vi "MFC_PID_flow_new.vi"() -> ()   [LabVIEW 2021]
uses:
  OdorSensorArray/labview 2016 code/osa_global_save2.vi
  <vilib>/Utility/file.llb/Read From Spreadsheet File (DBL).vi
  <vilib>/measure/NI_MABase.lvlib
panel:
  in  "Stair interval (s)":u32=20
  out "Error U3-2 A0":string
  out "PID / flow":cluster{"Value Read":dbl, "Value Read":dbl}(graph)
  in  "Dilusion_lj2_DAC1":dbl step=0.1 format="%.4f"
  out "elapsed time":string="00:00:00.000"
  in  "MFC_sequence":path
  out "Array Size":i32
  out "Udate Array from File":sgl[](array[numeric])
  out "Error  PID_Save":string
  out "error write":errorcluster
  in  "Save file":bool
  in  "save data folder":path
  out "appended path":path
  out "AIN0":dbl format="%.6f"
  out "MFC I/O":cluster{"Value Read":dbl, "Value Read":dbl}(graph)
  out "AIN2":dbl format="%.6f"
  out "AIN1":dbl format="%.6f"
  in  "DAC0_type":enum16{"functional", "fixed", "read"}(ring)
  out "Waveform Chart":dbl(graph)
  in  "DAC0_fixed":dbl step=0.1 format="%.4f"
  out "Error DAC1,B":string
  out "error read":errorcluster
  in  "Background_DAC1":dbl step=0.1 format="%.4f"
  in  "Update Interval (ms)":u32=20
  out "Error_DAC0":string
  in  "Function":u16(ring) items=["Sine Wave", "Triangle Wave", "Square Wave", "Sawtooth Wave"]
  in  "Min Voltage":dbl=0.5 min=0.0 max=5.0 step=0.1 format="%.2f"
  in  "Max Voltage":dbl=4.5 min=0.0 max=5.0 step=0.1 format="%.2f"
  in  "Frequency (Hz)":dbl=1.0 step=0.1 format="%.3f"
  in  "Stop":bool
  # "Updates DAC0 at the specified update interval in order to build time series waveforms.  The\nupdate interval is set to 20 ms by default, but can be set lower based on the execution times\ndiscussed in Section 3.1 of the U3 User's Guide.  Uses the first found U3.\n\nWith a software timed application such as this, you might be able to reduce timing jitter (caused\nby the operating system) by increasing the priority of this process (labview.exe) in Windows\nTask Manager."
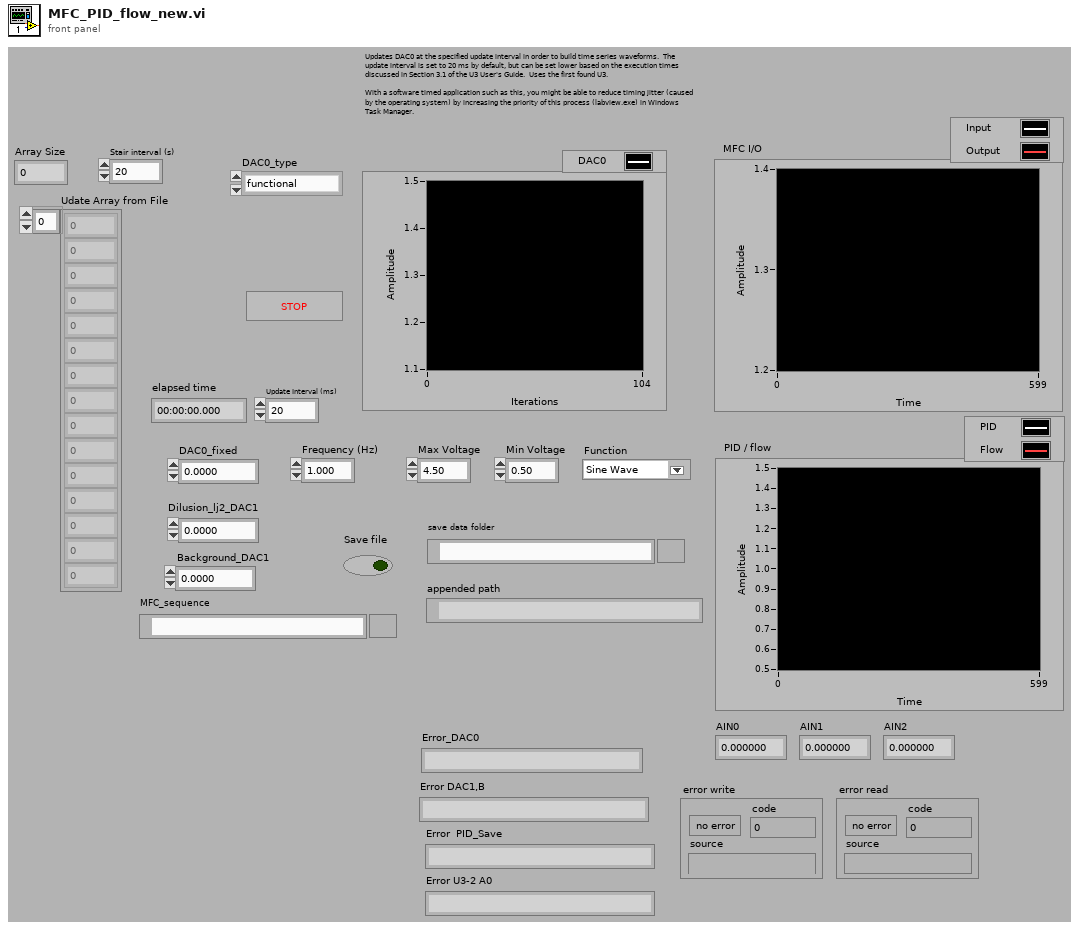
[diagram p1: front panel]
types:
  T1 = enum16{"open", "replace", "create", "open or create", "replace or create", "replace or create with confirmation"}
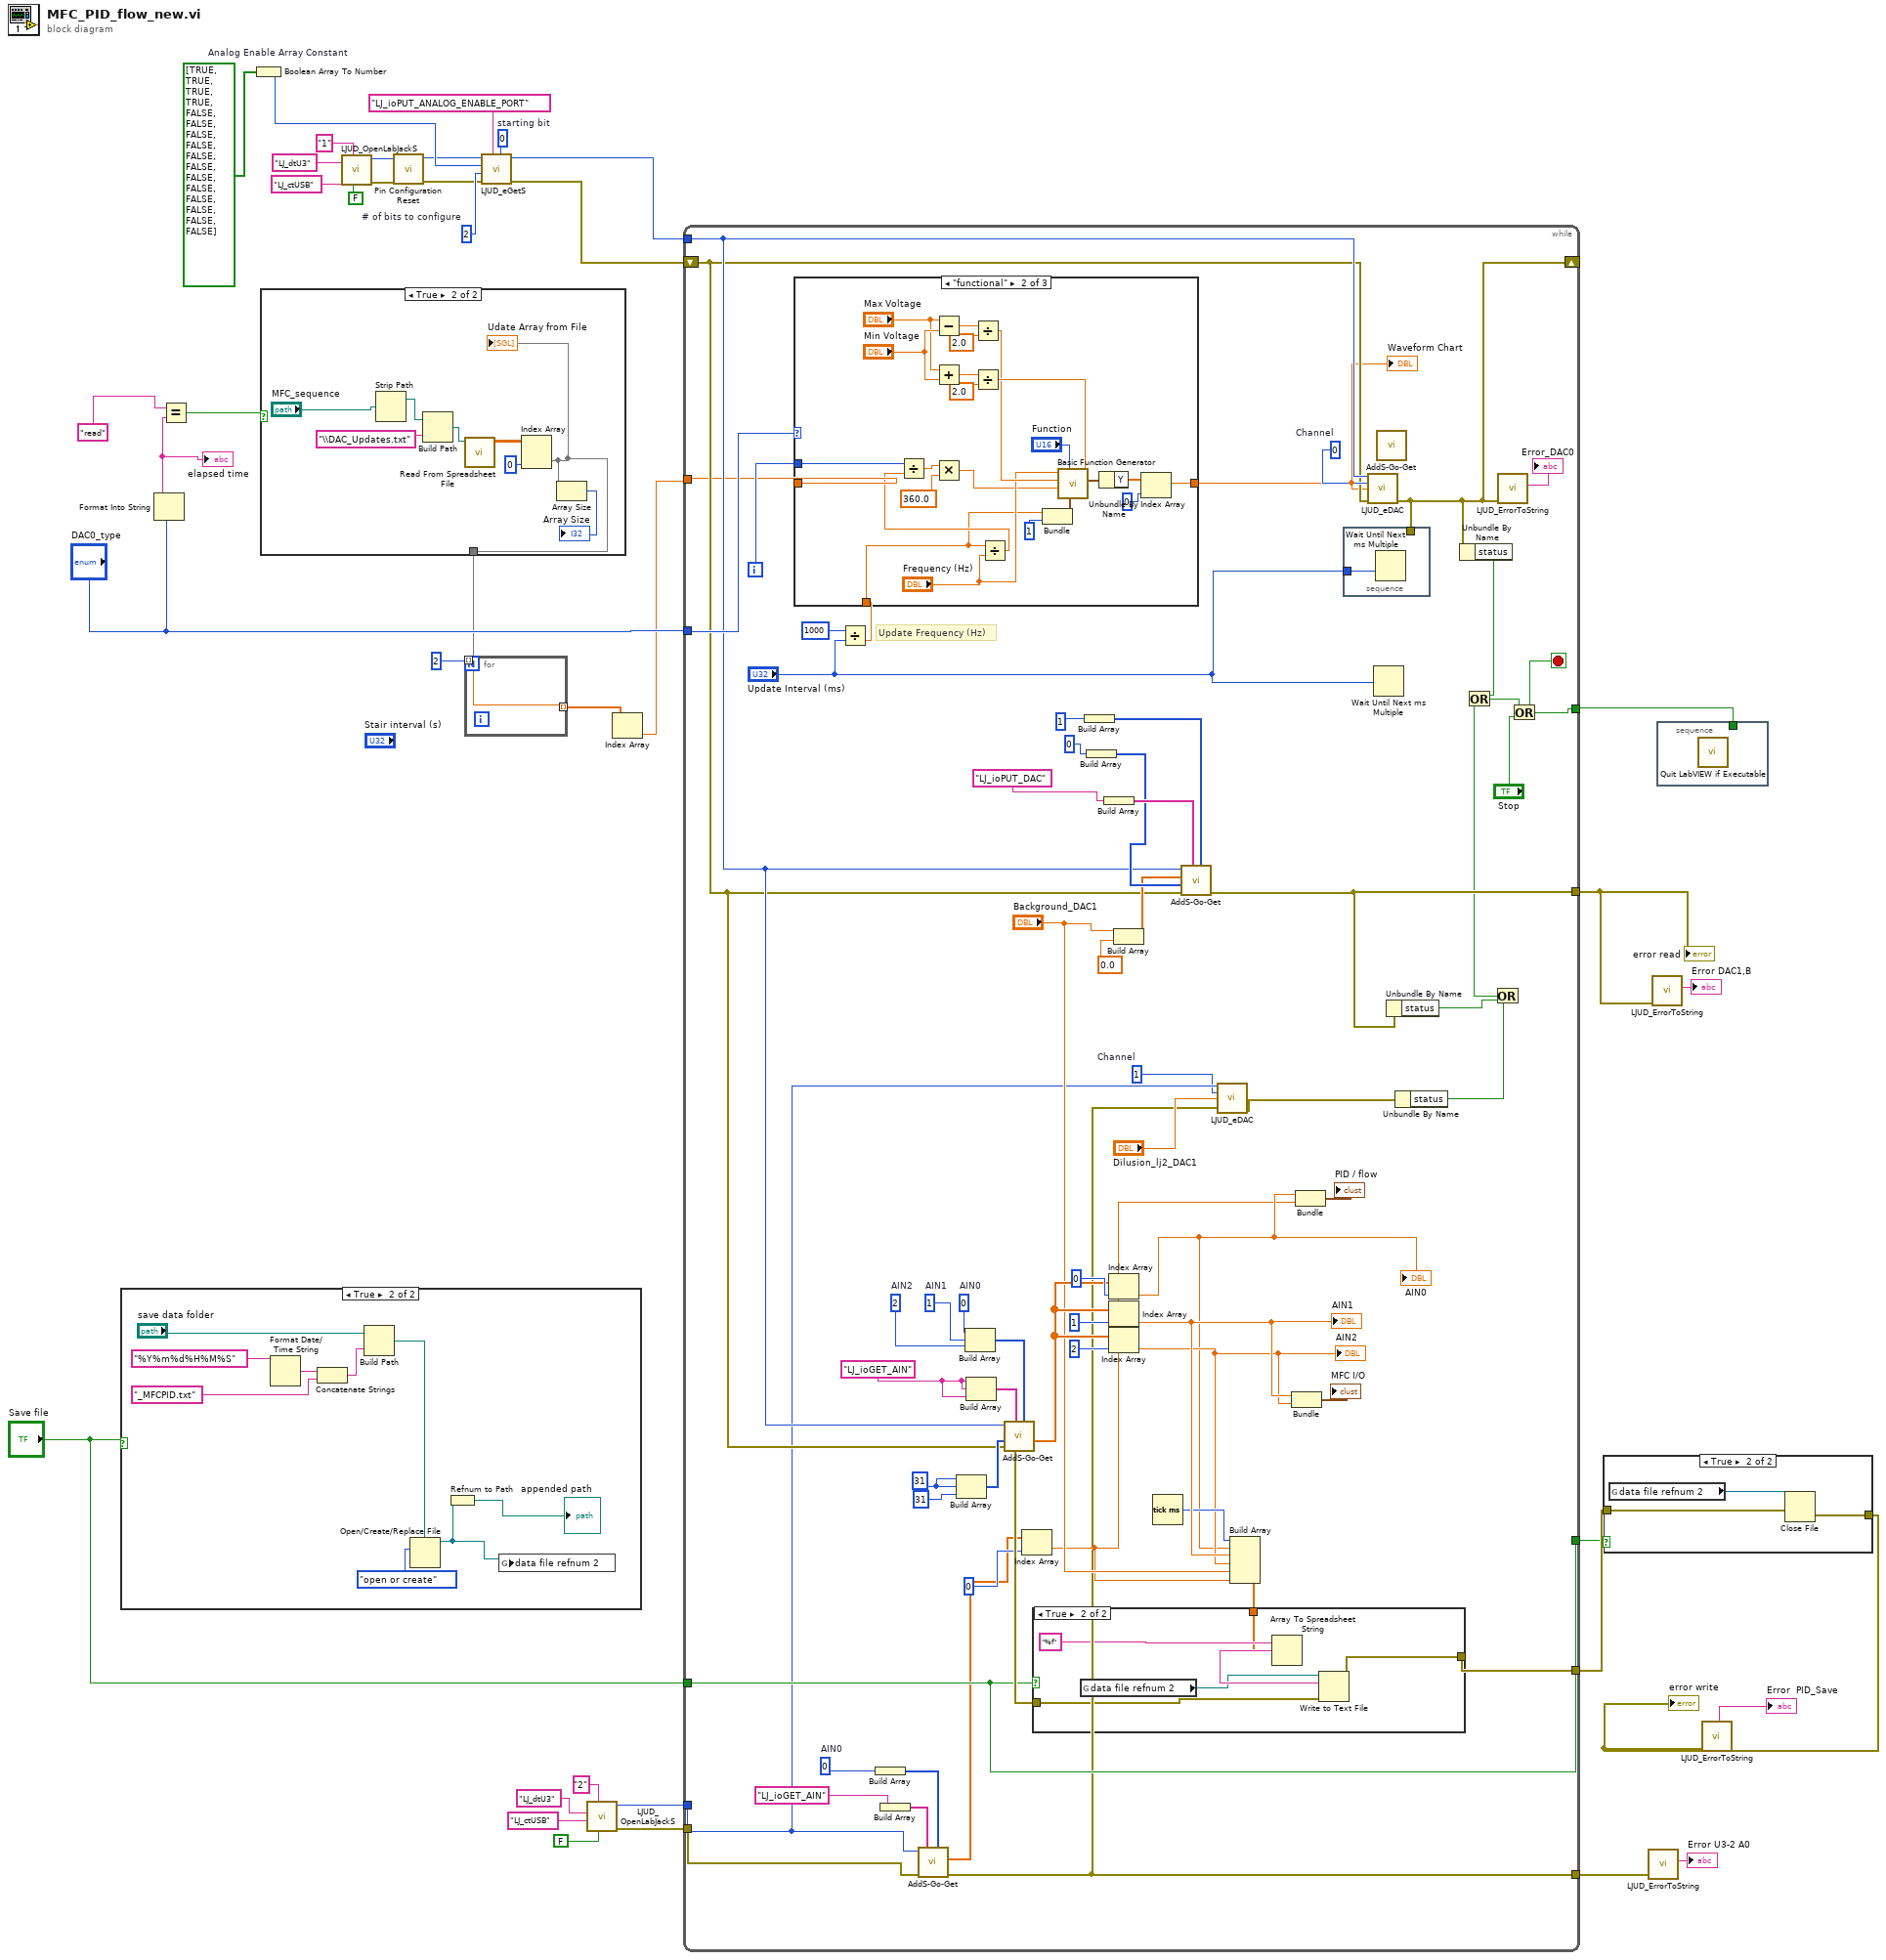
[diagram p0: block diagram]
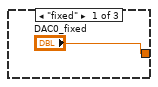
[diagram p6: hidden frame]
diagram:
  w27 = 2  # # of bits to configure
  w29 = 0  # starting bit
  w30 = bool[] [TRUE, TRUE, TRUE, TRUE, FALSE, FALSE, FALSE, FALSE, FALSE, FALSE, FALSE, FALSE, FALSE, FALSE, FALSE, FALSE]  # Analog Enable Array Constant
  n1 = case shown="True" "Save file" {
    frame False {
    }
    frame True {
      n2 = Format Date/Time String(time format string (%c)="%Y%m%d%H%M%S") -> (date/time string=w45:string)  [unwired: 2 in]
      n3 = Concatenate Strings(w45, "_MFCPID.txt") -> (w47:string)
      n4 = Build Path(base path="save data folder", name or relative path=w47) -> (appended path=w41:path)
      n5 = Open/Create/Replace File(file path (use dialog)=w41, operation (0:open)=T1."open or create") -> (refnum out=w40:refnum<file>)  [unwired: 4 in, 2 out]
      n6 = Refnum to Path(1:w40) -> (0:→"appended path":path)
      n7 = global write "osa_global_save2.vi" "data file refnum 2"(w40) -> ()
    }
  }
  n8 = Format Into String("DAC0_type") -> (resulting string=w13:string)  [unwired: 3 in, 1 out]
  "elapsed time" <- w13
  n9 = Equal?(x="read", y=w13) -> (x = y?=w16:bool)
  n10 = Boolean Array To Number(Boolean array=w30) -> (number=w26:u32)
  n11 = case shown="True" w16 {
    tunnel: [_ w49] -> w2
    frame False {
    }
    frame True {
      n12 = Strip Path(path="MFC_sequence") -> (stripped path=w51:path)  [unwired: 1 out]
      n13 = Build Path(base path=w51, name or relative path="\\DAC_Updates.txt" ("file path (dialog if empty)")) -> (appended path=w52:path)
      n14 = call-poly <vilib>:"Read From Spreadsheet File.vi"("file path (dialog if empty)"=w52) -> ("all rows"=w56:dbl[][])  [unwired: 6 in, 4 out]
      n15 = Index Array(array=w56, index (col)=0 ("disabled index (col)")) -> (element=w49:dbl[])  [unwired: 1 in]
      "Udate Array from File" <- w49
      n16 = Array Size(array=w49) -> (size(s)=→"Array Size":i32)
    }
  }
  n17 = call "LJUD_OpenLabJackS.vi"("FirstFound"=FALSE, "Address"="1" ("DeviceType"), "ConnectionType"="LJ_ctUSB", "DeviceType"="LJ_dtU3") -> ("error out"=w31:errorcluster, "Handle"=w32:i32)  [unwired: 5 in, 1 out]
  n18 = call "Pin Configuration Reset.vi"("error in"=w31, "Handle In"=w32) -> ("error out"=w24:errorcluster, "Handle Out"=w25:i32)  [unwired: 8 in]
  n19 = for {
    N: u32 2 ("x") -> [_]
    tunnel: [w57] -> w3 mode=indexing
    tunnel: w2 -> [w57] mode=indexing
  }
  n20 = call "LJUD_eGetS.vi"("Channel"=w29, "IOType"="LJ_ioPUT_ANALOG_ENABLE_PORT", "error in"=w24, "x1"=w27, "Value Write"=w26, "Handle In"=w25) -> ("error out"=w22:errorcluster, "Handle Out"=w23:i32)  [unwired: 3 in, 1 out]
  n21 = call "LJUD_OpenLabJackS.vi"("FirstFound"=FALSE, "Address"="2", "ConnectionType"="LJ_ctUSB", "DeviceType"="LJ_dtU3") -> ("error out"=w7:errorcluster, "Handle"=w8:i32)  [unwired: 5 in, 1 out]
  n22 = Index Array(array=w3) -> (element=w1:dbl)  [unwired: 1 in]
  n23 = while {
    tunnel: w23 -> [w83]
    shift-left: w22 -> [w82]
    shift-right: [w118] -> _
    tunnel: [w104] -> w39
    tunnel: [w107] -> w37
    tunnel: "DAC0_type" -> [w103]
    tunnel: w1 -> [w63]
    tunnel: [w79] -> w21
    tunnel: "Save file" -> [w77]
    tunnel: [w77] -> w19
    tunnel: w8 -> [w59]
    tunnel: w7 -> [w70]
    tunnel: [w60] -> w5
    i -> [w122]
    stop <- w104 stop-if-true
    w58 = 1  # Channel
    w73 = 0  # AIN0
    w89 = 2  # AIN2
    w85 = 31 ("AIN0")
    w94 = 1  # AIN1
    w93 = 0  # AIN0
    w86 = "LJ_ioGET_AIN" ("IOType")
    w119 = 0  # Channel
    # "Update Frequency (Hz)"
    n24 = Divide(x=u32 1000, y="Update Interval (ms)") -> (x/y=w116:dbl)
    n25 = case shown="\"functional\"" w103 {
      tunnel: w122 -> [_ w152 _]
      tunnel: ["DAC0_fixed" w132 w153] -> w64
      tunnel: w116 -> [_ w131 _]
      tunnel: w63 -> [_ _ w153]
      frame "fixed" {
      }
      frame "functional" {
        n26 = Subtract(x="Max Voltage", y="Min Voltage") -> (x-y=w149:dbl)
        n27 = Add(x="Max Voltage", y="Min Voltage") -> (x+y=w146:dbl)
        n28 = Divide(x=w149, y=2.0) -> (x/y=w141:dbl)
        n29 = Divide(x=w146, y=2.0) -> (x/y=w142:dbl)
        n30 = Divide(x=w131, y="Frequency (Hz)") -> (x/y=w151:dbl)
        n31 = Divide(x=w152, y=w151) -> (x/y=w150:dbl)
        n32 = Multiply(x=w150, y=360.0) -> (x*y=w138:dbl)
        n33 = Bundle(w131, 1) -> (w136:cluster{dbl, i32})  [unwired: 1 in]
        n34 = call <vilib>:"Basic Function Generator.vi"("offset"=w142, "sampling info"=w136, "signal type"="Function", "phase"=w138, "amplitude"=w141, "frequency"="Frequency (Hz)") -> ("signal out"=w135:waveform(dbl))  [unwired: 3 in, 2 out]
        n35 = Unbundle By Name(w135) -> ("Y"=w134:dbl[])
        n36 = Index Array(array=w134, index=0 ("Index")) -> (element=w132:dbl)
      }
      frame "read" {
      }
    }
    "Waveform Chart" <- w64
    n37 = Build Array(w73) -> (w74:i32[])
    n38 = Build Array("LJ_ioGET_AIN" ("IOType")) -> (w72:string[])
    n39 = call "AddS-Go-Get.vi"("Channels"=w74, "IOTypes"=w72, "error in"=w70, "Handle In"=w59) -> ("error out"=w60:errorcluster, "Values Read"=w66:dbl[])  [unwired: 5 in, 1 out]
    n40 = Build Array(w85, w85, 31 ("AIN1")) -> (w90:i32[])
    n41 = Build Array(w93, w94, w89) -> (w97:i32[])
    n42 = Build Array(w86, w86, w86) -> (w98:string[])
    n43 = call "AddS-Go-Get.vi"("Channels"=w97, "IOTypes"=w98, "error in"=w82, "x1"=w90, "Handle In"=w83) -> ("error out"=w80:errorcluster, "Values Read"=w78:dbl[])  [unwired: 4 in, 1 out]
    n44 = Index Array(array=w66, index=0 ("Index")) -> (element=w65:dbl)
    n45 = Build Array(1) -> (w114:i32[])
    n46 = Build Array(0) -> (w109:i32[])
    n47 = Build Array("LJ_ioPUT_DAC" ("IOType")) -> (w115:string[])
    n48 = Index Array(array=w78, index=0 ("Index")) -> (element=w68:dbl)
    "AIN0" <- w68
    n49 = Index Array(array=w78, index=1 ("Index")) -> (element=w87:dbl)
    "AIN1" <- w87
    n50 = Index Array(array=w78, index=2 ("Index")) -> (element=w81:dbl)
    "AIN2" <- w81
    n51 = Build Array("Background_DAC1", 0.0 ("Input Element")) -> (w102:dbl[])
    n52 = Tick Count (ms)() -> (millisecond timer value=w84:u32)
    n53 = call "AddS-Go-Get.vi"("Channels"=w114, "IOTypes"=w115, "error in"=w82, "x1"=w109, "Values Write"=w102, "Handle In"=w83) -> ("error out"=w107:errorcluster)  [unwired: 3 in, 2 out]
    n54 = call "LJUD_eDAC.vi"("Handle In"=w59, "Channel"=w58, "Voltage"="Dilusion_lj2_DAC1", "error in"=w60) -> ("error out"=w61:errorcluster)  [unwired: 10 in, 1 out]
    n55 = Build Array(w84, w68, w87, w81, "Background_DAC1", w65) -> (w76:dbl[])
    n56 = case shown="True" w77 {
      tunnel: w80 -> [w123 w128]
      tunnel: [w123 w127] -> w79
      tunnel: w76 -> [_ w124]
      frame False {
      }
      frame True {
        n57 = global read "osa_global_save2.vi" "data file refnum 2"() -> (w125:refnum<file>)
        n58 = Array To Spreadsheet String(array=w124, 3:"%f") -> (spreadsheet string=w126:string)  [unwired: 1 in]
        n59 = Write to Text File(file (use dialog)=w125, text=w126, error in=w128) -> (error out=w127:errorcluster)  [unwired: 1 in, 2 out]
      }
    }
    n60 = Bundle("Value Read"=w87, "Value Read"=w81) -> (→"MFC I/O":cluster{"Value Read":dbl, "Value Read":dbl})  [unwired: 1 in]
    n61 = Bundle("Value Read"=w68, "Value Read"=w65) -> (→"PID / flow":cluster{"Value Read":dbl, "Value Read":dbl})  [unwired: 1 in]
    n62 = call "LJUD_eDAC.vi"("Handle In"=w83, "Channel"=w119, "Voltage"=w64, "error in"=w82) -> ("error out"=w118:errorcluster)  [unwired: 10 in, 1 out]
    n63 = stacked-sequence {
      tunnel: "Update Interval (ms)" -> [w154]
      tunnel: w118 -> [_]
      frame #0 {
        n64 = Wait Until Next ms Multiple(millisecond multiple=w154) -> ()  [unwired: 1 out]
      }
    }
    n65 = Wait Until Next ms Multiple(millisecond multiple="Update Interval (ms)") -> ()  [unwired: 1 out]
    n66 = call "AddS-Go-Get.vi"() -> ()  [unwired: 9 in, 3 out]
    n67 = Unbundle By Name(w107) -> ("status"=w99:bool)
    n68 = Unbundle By Name(w61) -> ("status"=w100:bool)
    n69 = Unbundle By Name(w118) -> ("status"=w106:bool)
    n70 = Or(x=w100, y=w99) -> (x .or. y?=w101:bool)
    n71 = Or(x=w106, y=w101) -> (x .or. y?=w105:bool)
    n72 = call "LJUD_ErrorToString.vi"("error in"=w118) -> ("String"=→"Error_DAC0":string)  [unwired: 10 in]
    n73 = Or(x=w105, y="Stop") -> (x .or. y?=w104:bool)
  }
  "error read" <- w37
  n74 = case shown="True" w19 {
    tunnel: w21 -> [w155 w158]
    tunnel: [w155 w157] -> w17
    frame False {
    }
    frame True {
      n75 = global read "osa_global_save2.vi" "data file refnum 2"() -> (w156:refnum<file>)
      n76 = Close File(refnum=w156, error in=w158) -> (error out=w157:errorcluster)  [unwired: 1 out]
    }
  }
  "error write" <- w17
  n77 = call "LJUD_ErrorToString.vi"("error in"=w5) -> ("String"=→"Error U3-2 A0":string)  [unwired: 10 in]
  n78 = call "LJUD_ErrorToString.vi"("error in"=w37) -> ("String"=→"Error DAC1,B":string)  [unwired: 10 in]
  n79 = stacked-sequence {
    tunnel: w39 -> [_]
    frame #0 {
      n80 = call "Quit LabVIEW if Executable.vi"() -> ()  [unwired: 1 in]
    }
  }
  n81 = call "LJUD_ErrorToString.vi"("error in"=w17) -> ("String"=→"Error  PID_Save":string)  [unwired: 10 in]
